vi "RX Message.vi"(8 "error in (no error)":errorcluster, 11 "PID in":refnum<class "PID.lvclass">) -> (0 "error out":errorcluster, 2 "String":string, 3 "PID out":refnum<class "PID.lvclass">)   [LabVIEW 2011, in "PID.lvclass"]
uses:
  PID.lvclass
  PID.lvclass/PID.ctl
panel:
  out "x-y":dbl format="%#_6p"
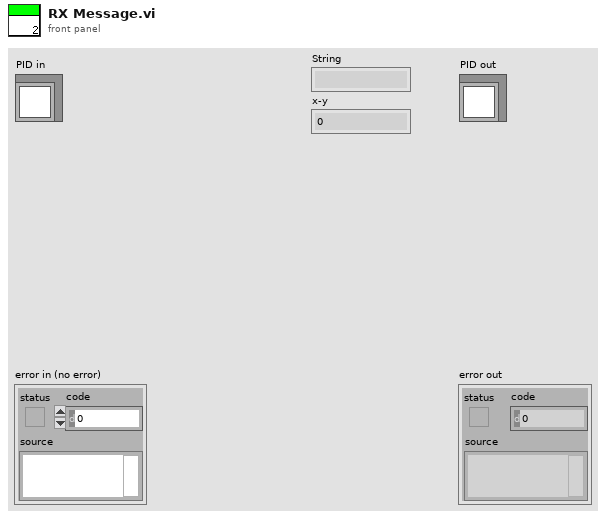
[diagram p1: front panel]
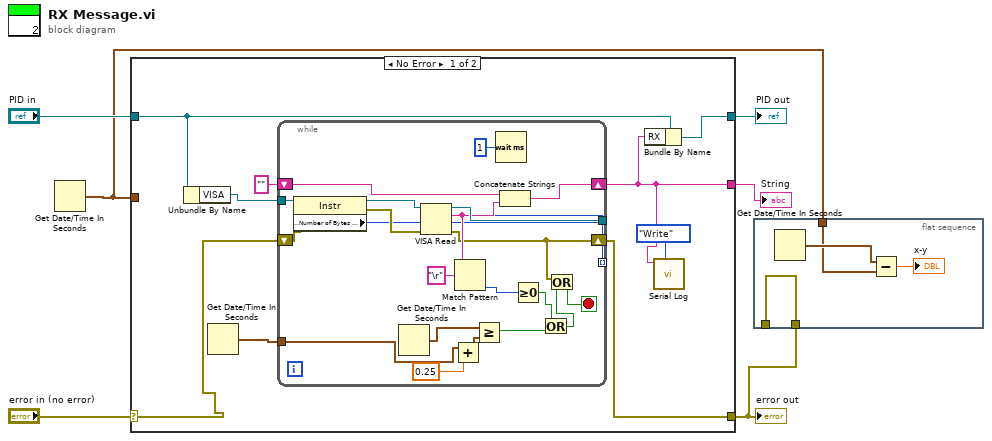
[diagram p0: block diagram]
diagram:
  n1 = Get Date/Time In Seconds() -> (seconds since 1Jan1904=w1:timestamp)
  n2 = case shown="No Error" "error in (no error)" {
    selector: "error in (no error)" -> [w8 w38]
    tunnel: [w7 w38] -> w2
    tunnel: [w9 w37] -> w4
    tunnel: "PID in" -> [w10 w37]
    tunnel: [w11 _] -> w3
    tunnel: w1 -> [_ _]
    frame No Error {
      n3 = Unbundle By Name(w10) -> ("VISA"=w13:refnum<visa-resource-name>)
      n4 = Get Date/Time In Seconds() -> (seconds since 1Jan1904=w14:timestamp)
      n5 = while {
        tunnel: w13 -> [w36]
        shift-right: [w31] -> w11
        shift-left: "" -> [w30]
        tunnel: [w29] -> _
        shift-right: [w17] -> w7
        shift-left: w8 -> [w28]
        tunnel: [w26] -> _ mode=indexing
        tunnel: w14 -> [w24]
        stop <- w16 stop-if-true
        n6 = property class="Instr"(reference=w36, error in=w28) -> (reference out=w35:refnum<visa-resource-name>, error out=w34:errorcluster, "Serial Settings:Number of Bytes at Serial Port"=w26:u32)
        n7 = Get Date/Time In Seconds() -> (seconds since 1Jan1904=w25:timestamp)
        n8 = VISA Read(VISA resource name=w35, byte count=w26, error in (no error)=w34) -> (VISA resource name out=w29:refnum<visa-resource-name>, read buffer=w27:string, error out=w17:errorcluster)  [unwired: 1 out]
        n9 = Add(x=w24, y=0.25) -> (x+y=w22:timestamp)
        n10 = Match Pattern(string=w27, regular expression="\r") -> (offset past match=w32:i32)  [unwired: 1 in, 3 out]
        n11 = Greater Or Equal?(x=w25, y=w22) -> (x >= y?=w20:bool)
        n12 = Wait (ms)(milliseconds to wait=u32 1) -> ()  [unwired: 1 out]
        n13 = Concatenate Strings(w30, w27) -> (w31:string)
        n14 = Greater Or Equal To 0?(x=w32) -> (x >= 0?=w21:bool)
        n15 = Or(x=w21, y=w20) -> (x .or. y?=w18:bool)
        n16 = Or(x=w17, y=w18) -> (x .or. y?=w16:bool)
      }
      n17 = Bundle By Name(cluster=w10, "RX"=w11) -> (w9:refnum<class "PID.lvclass">)
      n18 = call "Serial Log.vi"("State"=enum16{"Init", "Write", "Read"}."Write", "String"=w11) -> ()  [unwired: 7 in, 3 out]
    }
    frame Error {
    }
  }
  "error out" <- w2
  "PID out" <- w4
  "String" <- w3
  n19 = flat-sequence {
    tunnel: [w42] -> _
    tunnel: w2 -> [w42]
    tunnel: w1 -> [w40]
    frame #0 {
      n20 = Get Date/Time In Seconds() -> (seconds since 1Jan1904=w41:timestamp)
      n21 = Subtract(x=w41, y=w40) -> (x-y=→"x-y":dbl)
    }
  }
